vi "ZDelay_node_test.vi"() -> ()   [LabVIEW 2018]
uses:
  Tracker.lvlib
panel:
  out "Array 2":dbl[](array[numeric])
  out "Array":dbl[](array[numeric])
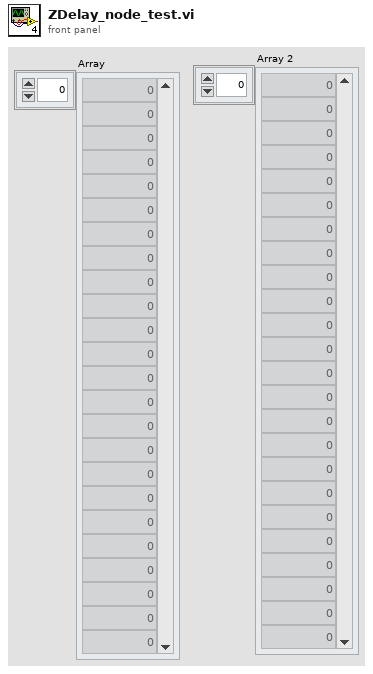
[diagram p1: front panel]
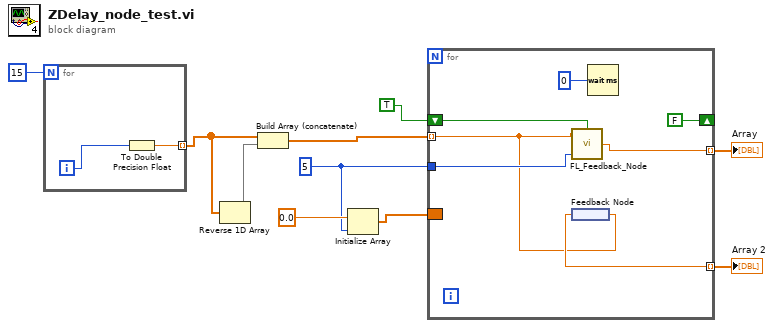
[diagram p0: block diagram]
diagram:
  w4 = 5 ("Buffer length, samples")
  n1 = for {
    N: 15 -> [_]
    tunnel: [w11] -> w3 mode=indexing
    i -> [w12]
    n2 = To Double Precision Float(number=w12) -> (double precision float=w11:dbl)
  }
  n3 = Reverse 1D Array(array=w3) -> (reversed array=w1:dbl[])
  n4 = Build Array (concatenate)(w3, w1) -> (w2:dbl[])
  n5 = Initialize Array(0.0, w4) -> (w5:dbl[])
  n6 = for {
    tunnel: w2 -> [w14] mode=indexing
    shift-right: [FALSE ("Reset buffer")] -> _
    shift-left: TRUE ("Reset buffer") -> [w15]
    tunnel: [w13] -> w8 mode=indexing
    border: w5 -> [_]
    tunnel: [w17] -> w7 mode=indexing
    tunnel: w4 -> [w16]
    n7 = call "FL_Feedback_Node.vi"("Reset Node"=w15, "Delay"=w16, "Input X"=w14) -> ("Delayed X"=w13:dbl)  [unwired: 1 in]
    n8 = feedback-in #1(w14) -> ()
    n9 = feedback #1() -> (w17:dbl)
    n10 = Wait (ms)(milliseconds to wait=u32 0) -> ()  [unwired: 1 out]
  }
  "Array" <- w8
  "Array 2" <- w7
